vi "Tell Self.vi"(4 "Priority":bool, 7 "Actor in":refnum<class "Actor.lvclass">, 10 "Msg":refnum<class "Msg.lvclass">) -> (0 "Error out":errorcluster)   [LabVIEW 2025, in "jettl.lvlib"]
uses:
  jettl.lvlib
  Relation.ctl
  Teller/Teller.lvlib
  Actor/Actor.lvclass
  Transport/Transport/Transport.lvclass
  Msg/Msg.lvclass
  Attributes/Attributes/Attributes.lvclass
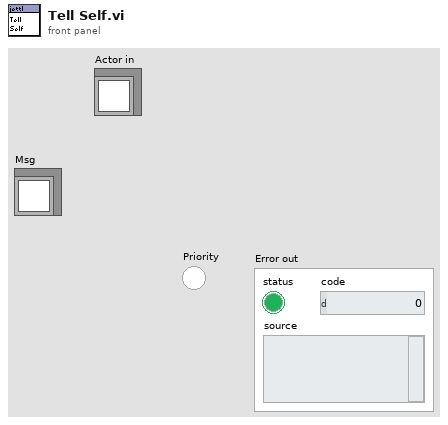
[diagram p1: front panel]
types:
  T1 = typedef "jettl.lvlib/Relation.ctl" = enum16{"Self", "Parent", "Child"}
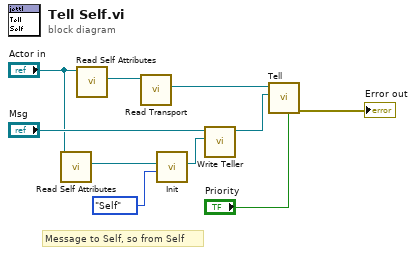
[diagram p0: block diagram]
diagram:
  # "Message to Self, so from Self"
  n1 = call-dynamic "Read Self Attributes.vi"("Actor in"="Actor in") -> ("Self Attributes"=w6:refnum<class "Attributes.lvclass">)  [unwired: 10 in]
  n2 = call-dynamic "Read Self Attributes.vi"("Actor in"="Actor in") -> ("Self Attributes"=w8:refnum<class "Attributes.lvclass">)  [unwired: 10 in]
  n3 = call-dynamic "Read Transport.vi"("Attributes in"=w8) -> ("Transport"=w4:refnum<class "Transport.lvclass">)  [unwired: 10 in]
  n4 = call "Init.vi"("Relation"=Relation."Self", "Self Attributes"=w6) -> ("Teller"=w7:refnum<class "Teller.lvclass">)  [unwired: 9 in]
  n5 = call-dynamic "Write Teller.vi"("Teller"=w7, "Msg in"="Msg") -> ("Msg out"=w3:refnum<class "Msg.lvclass">)  [unwired: 9 in]
  n6 = call-dynamic "Tell.vi"("Priority"="Priority", "Msg"=w3, "Transport in"=w4) -> ("Error out"=→"Error out":errorcluster)  [unwired: 8 in]
